vi "Measurement Parameter.vi"(8 "error in (no error)":errorcluster, 10 "Meas Parameter":T1, 11 "BK-Precision in":refnum<class "BK-Precision.lvclass">) -> (0 "error out":errorcluster, 2 "Value":dbl, 3 "BK-Precision out":refnum<class "BK-Precision.lvclass">)   [LabVIEW 2021, in "DC PWS.lvlib" / "BK-Precision.lvclass"]
uses:
  BK-Precision.lvclass
  BK-Precision.lvclass/BK-Precision.ctl
  <instrlib>/BK Precision 911X Series/BK Precision 911X Series.lvlib
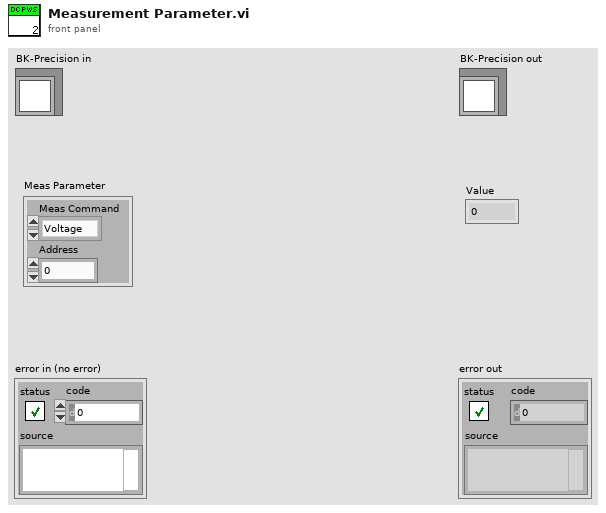
[diagram p1: front panel]
types:
  T1 = cluster{"Meas Command":enum16{"Voltage", "Current", "Power"}, "Address":dbl}
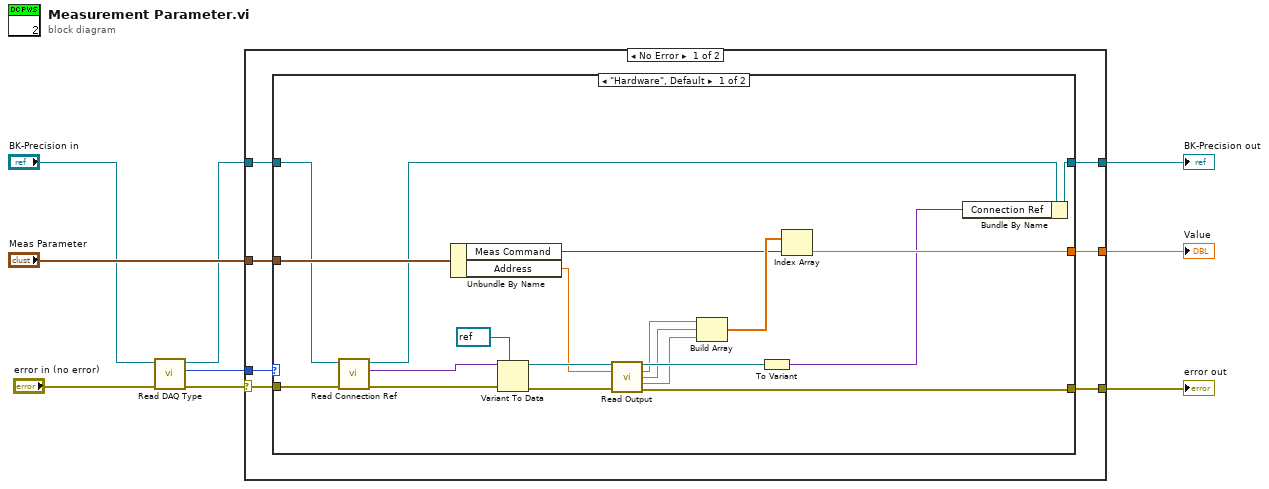
[diagram p0: block diagram]
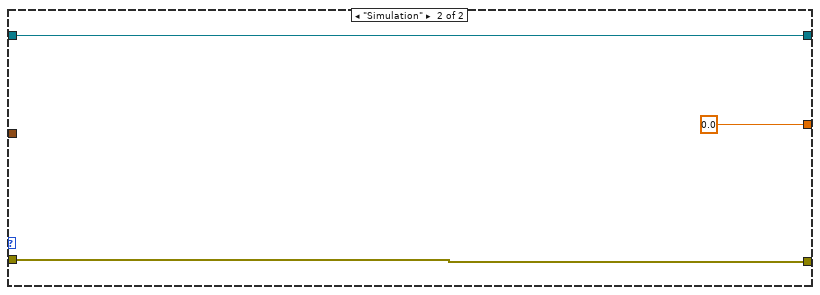
[diagram p2: hidden frame]
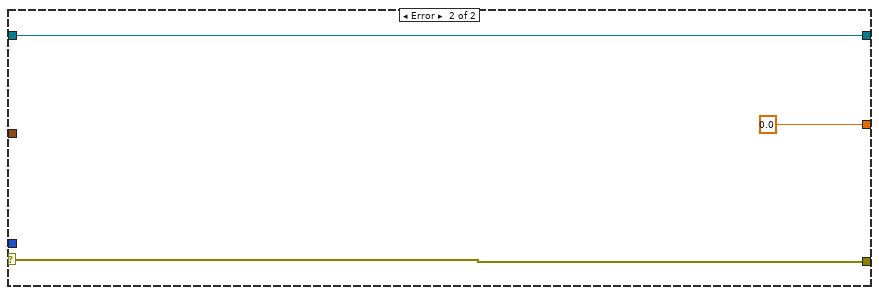
[diagram p3: hidden frame]
diagram:
  n1 = call "Read DAQ Type.vi"("error in (no error)"="error in (no error)", "BK-Precision in"="BK-Precision in") -> ("error out"=w8:errorcluster, "Type"=w7:enum16{"Hardware", "Simulation"}, "BK-Precision out"=w1:refnum<class "BK-Precision.lvclass">)  [unwired: 7 in]
  n2 = case shown="No Error" w8 {
    selector: w8 -> [w14 w41]
    tunnel: w7 -> [w16 _]
    tunnel: w1 -> [w15 w42]
    tunnel: [w13 w42] -> w6
    tunnel: "Meas Parameter" -> [w12 _]
    tunnel: [w11 w41] -> w4
    tunnel: [w10 0.0 ("Actual Power Level (W)")] -> w3
    frame No Error {
      n3 = case shown="\"Hardware\", Default" w16 {
        tunnel: w15 -> [w18 w39]
        tunnel: w14 -> [w36 w38]
        tunnel: [w28 w39] -> w13
        tunnel: w12 -> [w31 _]
        tunnel: [w26 w38] -> w11
        tunnel: [w20 0.0 ("Actual Power Level (W)")] -> w10
        frame "Hardware", Default {
          n4 = call "Read Connection Ref.vi"("error in (no error)"=w36, "BK-Precision in"=w18) -> ("error out"=w35:errorcluster, "Conn Ref"=w34:variant, "BK-Precision out"=w17:refnum<class "BK-Precision.lvclass">)  [unwired: 7 in]
          n5 = Unbundle By Name(w31) -> ("Meas Command"=w21:enum16{"Voltage", "Current", "Power"}, "Address"=w30:dbl)
          n6 = Variant To Data(error in=w35, type=refnum<visa-resource-name> refnum ("VISA resource name"), Variant=w34) -> (data=w32:refnum<visa-resource-name>, error out=w29:errorcluster)
          n7 = call <instrlib>:"Read Output.vi"("VISA resource name"=w32, "Address (0)"=w30, "error in (no error)"=w29) -> ("VISA resource name out"=w27:refnum<visa-resource-name>, "Actual Voltage Level (V)"=w25:dbl, "Actual Current Level (A)"=w24:dbl, "Actual Power Level (W)"=w23:dbl, "error out"=w26:errorcluster)  [unwired: 7 in, 1 out]
          n8 = Build Array(w25, w24, w23) -> (w22:dbl[])
          n9 = To Variant(anything=w27) -> (Variant=w19:variant)
          n10 = Index Array(array=w22, index=w21) -> (element=w20:dbl)
          n11 = Bundle By Name(cluster=w17, "Connection Ref"=w19) -> (w28:refnum<class "BK-Precision.lvclass">)
        }
        frame "Simulation" {
        }
      }
    }
    frame Error {
    }
  }
  "error out" <- w4
  "BK-Precision out" <- w6
  "Value" <- w3
